vi "Write.vi"(10 "Variant":variant, 11 "Variant in":refnum<class "Variant.lvclass">) -> (3 "Variant out":refnum<class "Variant.lvclass">)   [LabVIEW 2020, in "Data.lvlib" / "Variant.lvclass"]
doc: "Write Variant."
uses:
  Variant.lvclass
  Variant.lvclass/Variant.ctl
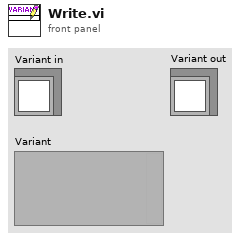
[diagram p1: front panel]
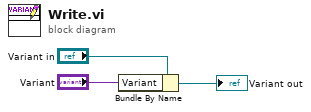
[diagram p0: block diagram]
diagram:
  n1 = Bundle By Name(cluster="Variant in", "Variant"="Variant") -> (→"Variant out":refnum<class "Variant.lvclass">)
